vi "CUNNINGHAM_Final-Project_Metal_Foam_Testing.vi"() -> ()   [LabVIEW 2010]
uses:
  <vilib>/Utility/error.llb/DialogType.ctl
  <vilib>/DAQmx/write.llb/DAQmx Write (Analog DBL 1Chan 1Samp).vi
  <vilib>/DAQmx/read.llb/DAQmx Read (Analog Wfm 1Chan NSamp).vi
  <vilib>/DAQmx/read.llb/DAQmx Read (Counter DBL 1Chan 1Samp).vi
  <vilib>/DAQmx/create/channels.llb/DAQmx Create Channel (CI-Frequency).vi
  <vilib>/DAQmx/create/channels.llb/DAQmx Create Channel (AI-Voltage-Basic).vi
  <vilib>/DAQmx/configure/timing.llb/DAQmx Timing (Sample Clock).vi
  <vilib>/DAQmx/create/channels.llb/DAQmx Create Channel (AO-Voltage-Basic).vi
  <vilib>/Utility/file.llb/Write To Spreadsheet File (string).vi
  <vilib>/Utility/file.llb/Write To Spreadsheet File (DBL).vi
  <vilib>/daqmx/miscellaneous.llb/DAQmx Fill In Error Info.vi
  <vilib>/Analysis/NI_AALBase.lvlib
panel:
  out "Collected Data":cluster{"mean":dbl, "data":dbl}[](graph)
  in  "Maximum Value":dbl=10.0 caption="Maximum Voltage to Blower" min=0.0 max=10.0 format="%0.2f"
  in  "Minimum Value":dbl caption="Minimum Voltage to Blower" min=0.0 max=10.0 format="%0.2f"
  out "Current Air Flow Speed (fpm)":dbl
  out "Current Pressure Drop (Pa)":dbl
  out "Frequency (Hz)":dbl format="%0.9f"
  out "Measurement":waveform(dbl)(graph)
  in  "Hold Time(ms)":u32=3000
  in  "Divisions for Air Flow Sweep":u8=5
  in  "Highest Voltage to Blower":dbl=3.3 min=0.0 max=10.0 format="%0.2f"
  in  "Staring Voltage to Blower":dbl=1.3 caption="Starting/Lowest Voltage to Blower" min=0.0 max=10.0 format="%0.2f"
  in  "Physical Channel":tag="Dev1/ao0" caption="AO Physical Channel Output"
  out "Voltage Output":dbl(slide)=1.0 scale=-10.0..9.995 scale format="%.3f"
  in  "AI Maximum Value":dbl=5.0 format="%0.2f"
  in  "AI Minimum Value":dbl format="%0.2f"
  in  "Rate":dbl=1000.0 caption="Sample Rate (Hz)" format="%0.0f"
  in  "Samples per Channel":i32=1000
  in  "Physical Channel":tag="Dev1/ai0" caption="AI Physical Channel Input"
  in  "Minimum Value (Hz)":dbl=1.192093 format="%0.6f"
  in  "Maximum Value (Hz)":dbl=10000000.0 format="%0.6f"
  in  "Edge":i32(ring)=10280 items=["Rising"=10280, "Falling"=10171]
  in  "Counter(s)":tag="Dev1/ctr0" caption="Frequency Physical Channel"
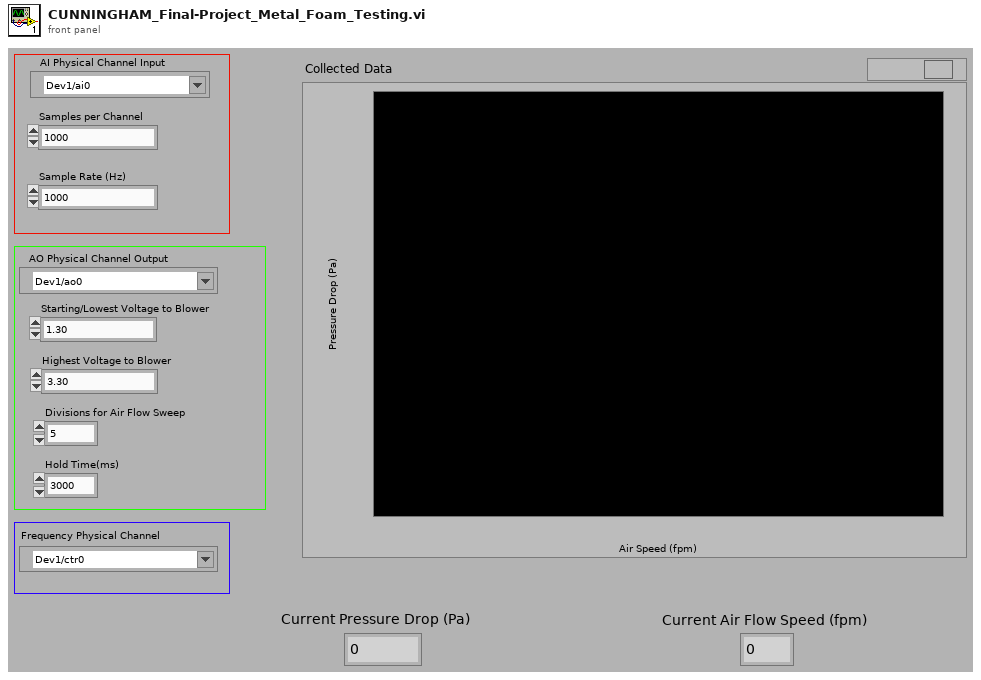
[diagram p1: front panel]
types:
  T1 = typedef "DialogType.ctl" = u16
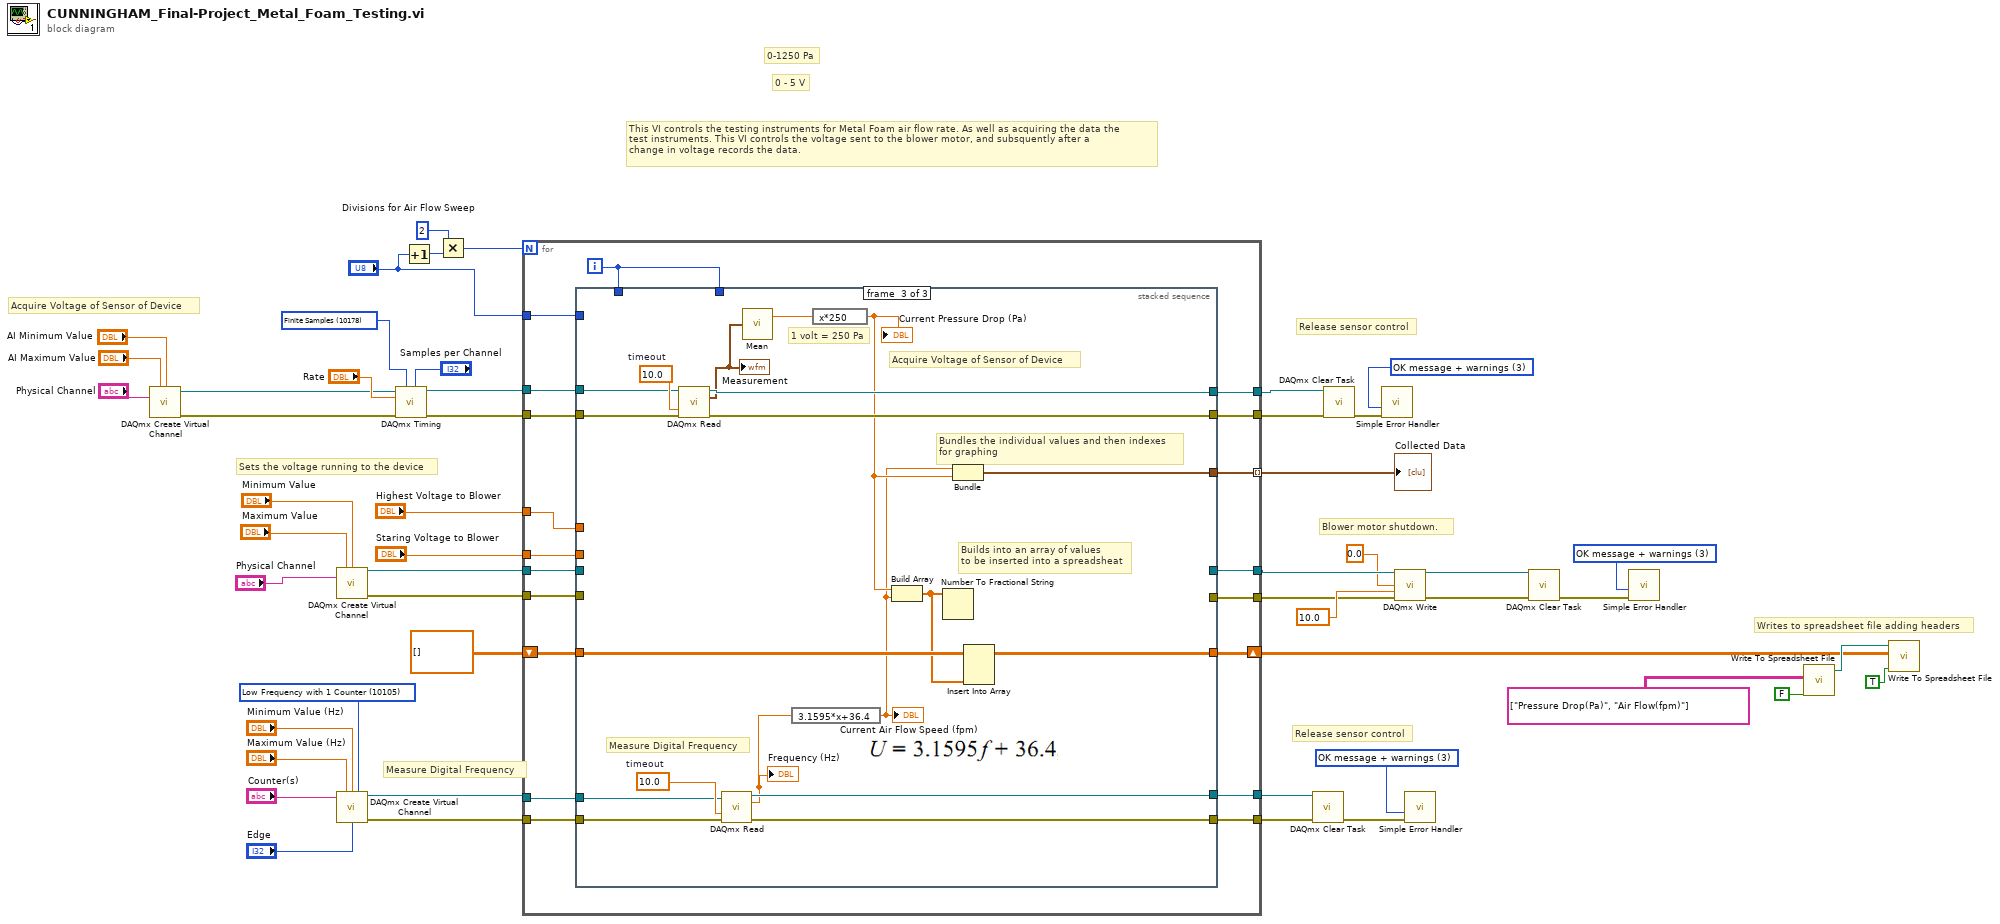
[diagram p0: block diagram]
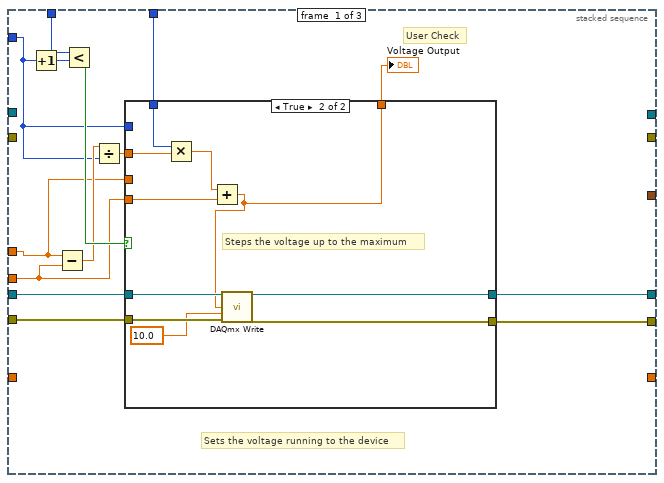
[diagram p2: hidden frame]
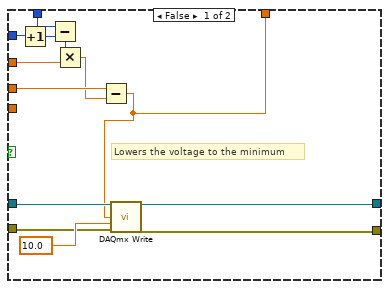
[diagram p3: hidden frame]
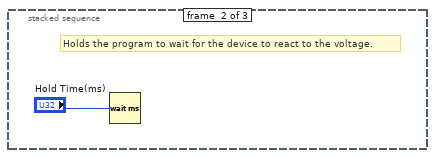
[diagram p4: hidden frame]
diagram:
  w33 = T1 3 items=["no dialog", "OK message", "continue or stop message", "OK message + warnings", "continue/stop + warnings"] ("type of dialog (OK msg:1)")
  w2 = 10178 items=["Finite Samples"=10178, "Continuous Samples"=10123] ("sample mode")
  w44 = T1 3 items=["no dialog", "OK message", "continue or stop message", "OK message + warnings", "continue/stop + warnings"] ("type of dialog (OK msg:1)")
  w49 = 10105 items=["Low Frequency with 1 Counter"=10105, "High Frequency with 2 Counters"=10157, "Large Range with 2 Counters"=10205] ("measurement method")
  w50 = T1 3 items=["no dialog", "OK message", "continue or stop message", "OK message + warnings", "continue/stop + warnings"] ("type of dialog (OK msg:1)")
  # "Writes to spreadsheet file adding headers"
  # "Release sensor control"
  # "Release sensor control"
  # "Sets the voltage running to the device"
  # "0 - 5 V"
  # "0-1250 Pa"
  # "Acquire Voltage of Sensor of Device"
  # "This VI controls the testing instruments for Metal Foam air flow rate. As well as acquiring the data the\ntest instruments. This VI controls the voltage sent to the blower motor, and subsquently after a\nchange in voltage records the data."
  # "Measure Digital Frequency"
  # "Blower motor shutdown."
  n1 = call-poly <vilib>:"DAQmx Create Virtual Channel.vi"("maximum value"="AI Maximum Value", "minimum value"="AI Minimum Value", "physical channels"="Physical Channel") -> ("task out"=w37:refnum<k21>, "error out"=w40:errorcluster)  [unwired: 11 in]
  n2 = call-poly <vilib>:"DAQmx Create Virtual Channel.vi"("maximum value"="Maximum Value", "minimum value"="Minimum Value", "physical channels"="Physical Channel") -> ("task out"=w32:refnum<k21>, "error out"=w30:errorcluster)  [unwired: 11 in]
  n3 = call-poly <vilib>:"DAQmx Create Virtual Channel.vi"("maximum value"="Maximum Value (Hz)", "minimum value"="Minimum Value (Hz)", "measurement method"=w49, "counter"="Counter(s)", "starting edge"="Edge") -> ("task out"=w29:refnum<k21>, "error out"=w28:errorcluster)  [unwired: 9 in]
  n4 = call-poly <vilib>:"DAQmx Timing.vi"("task/channels in"=w37, "sample mode"=w2, "samples per channel"="Samples per Channel", "rate"="Rate", "error in"=w40) -> ("task out"=w35:refnum<k21>, "error out"=w34:errorcluster)  [unwired: 9 in]
  n5 = Increment(x="Divisions for Air Flow Sweep") -> (x+1=w10:u8)
  n6 = Multiply(x=u8 2, y=w10) -> (x*y=w14:u8)
  n7 = for {
    N: w14 -> [_]
    tunnel: w35 -> [w66]
    tunnel: w34 -> [w65]
    tunnel: w32 -> [w70]
    tunnel: [w69] -> w21
    tunnel: [w68] -> w22
    tunnel: w30 -> [w67]
    tunnel: w29 -> [w64]
    tunnel: w28 -> [w63]
    tunnel: [w62] -> w27
    tunnel: [w61] -> w26
    tunnel: [w60] -> w25
    tunnel: [w59] -> w9
    tunnel: "Staring Voltage to Blower" -> [w58]
    tunnel: "Divisions for Air Flow Sweep" -> [w57]
    tunnel: "Highest Voltage to Blower" -> [w56]
    shift-right: [w53] -> w4
    shift-left: dbl[][] [] -> [w54]
    tunnel: [w52] -> w3 mode=indexing
    i -> [w55]
    n8 = stacked-sequence {
      tunnel: w70 -> [w84 _ _]
      tunnel: [w83 _ _] -> w69
      tunnel: [w82 _ _] -> w68
      tunnel: w67 -> [w81 _ _]
      tunnel: w66 -> [_ _ w126]
      tunnel: w65 -> [_ _ w123]
      tunnel: w64 -> [_ _ w121]
      tunnel: w63 -> [_ _ w120]
      tunnel: [_ _ w119] -> w62
      tunnel: [_ _ w118] -> w61
      tunnel: [_ _ w125] -> w60
      tunnel: [_ _ w124] -> w59
      tunnel: w58 -> [w71 _ _]
      tunnel: w57 -> [w73 _ _]
      tunnel: w56 -> [w72 _ _]
      tunnel: w55 -> [w80 _ _]
      tunnel: w55 -> [w78 _ _]
      tunnel: w54 -> [_ _ w114]
      tunnel: [_ _ w112] -> w53
      tunnel: [_ _ w111] -> w52
      frame #0 {
        # "User Check"
        # "Sets the voltage running to the device"
        n9 = Increment(x=w73) -> (x+1=w74:u8)
        n10 = Subtract(x=w72, y=w71) -> (x-y=w76:dbl)
        n11 = Less?(x=w78, y=w74) -> (x < y?=w77:bool)
        n12 = Divide(x=w76, y=w73) -> (x/y=w79:dbl)
        n13 = case shown="True" w77 {
          tunnel: w84 -> [w93 w107]
          tunnel: [w96 w106] -> w83
          tunnel: [w95 w105] -> w82
          tunnel: w81 -> [w94 w104]
          tunnel: w80 -> [w87 w102]
          tunnel: w79 -> [w92 w101]
          tunnel: w71 -> [_ w100]
          tunnel: w73 -> [w85 _]
          tunnel: w72 -> [w90 _]
          tunnel: [w88 w98] -> w75
          frame False {
            # "Lowers the voltage to the minimum"
            n14 = Increment(x=w85) -> (x+1=w86:u8)
            n15 = Subtract(x=w87, y=w86) -> (x-y=w91:i32)
            n16 = Multiply(x=w91, y=w92) -> (x*y=w89:dbl)
            n17 = Subtract(x=w90, y=w89) -> (x-y=w88:dbl)
            n18 = call-poly <vilib>:"DAQmx Write.vi"("task/channels in"=w93, "data"=w88, "timeout"=10.0, "error in"=w94) -> ("task out"=w96:refnum<k21>, "error out"=w95:errorcluster)  [unwired: 9 in, 1 out]
          }
          frame True {
            # "Steps the voltage up to the maximum"
            n19 = Multiply(x=w102, y=w101) -> (x*y=w99:dbl)
            n20 = Add(x=w99, y=w100) -> (x+y=w98:dbl)
            n21 = call-poly <vilib>:"DAQmx Write.vi"("task/channels in"=w107, "data"=w98, "timeout"=10.0, "error in"=w104) -> ("task out"=w106:refnum<k21>, "error out"=w105:errorcluster)  [unwired: 9 in, 1 out]
          }
        }
        "Voltage Output" <- w75
      }
      frame #1 {
        # "Holds the program to wait for the device to react to the voltage."
        n22 = Wait (ms)(milliseconds to wait="Hold Time(ms)") -> ()  [unwired: 1 out]
      }
      frame #2 {
        w122 = 10.0  # timeout
        w127 = 10.0  # timeout
        # "1 volt = 250 Pa"
        # "Bundles the individual values and then indexes\nfor graphing"
        # "Builds into an array of values \nto be inserted into a spreadsheat"
        # "Acquire Voltage of Sensor of Device"
        # "Measure Digital Frequency"
        n23 = call-poly <vilib>:"DAQmx Read.vi"("task/channels in"=w126, "timeout"=w127, "error in"=w123) -> ("task out"=w125:refnum<k21>, "data"=w117:waveform(dbl), "error out"=w124:errorcluster)  [unwired: 10 in]
        "Measurement" <- w117
        n24 = call-poly <vilib>:"DAQmx Read.vi"("task/channels in"=w121, "timeout"=w122, "error in"=w120) -> ("task out"=w119:refnum<k21>, "data"=w115:dbl, "error out"=w118:errorcluster)  [unwired: 10 in]
        "Frequency (Hz)" <- w115
        n25 = call <vilib>:"Mean.vi"("X"=w117) -> ("mean"=w116:dbl)  [unwired: 1 out]
        n26 = expression code="3.1595*x+36.4"(w115) -> (w109:dbl)
        "Current Air Flow Speed (fpm)" <- w109
        n27 = expression code="x*250"(w116) -> (w110:dbl)
        "Current Pressure Drop (Pa)" <- w110
        n28 = Build Array(w110, w109) -> (w113:dbl[])
        n29 = Number To Fractional String(number=w113) -> ()  [unwired: 3 in, 1 out]
        n30 = Bundle("data"=w109, "mean"=w110) -> (w111:cluster{"data":dbl, "mean":dbl})  [unwired: 1 in]
        n31 = Insert Into Array(array=w114, new element=w113) -> (w112:dbl[][])  [unwired: 2 in]
      }
    }
  }
  "Collected Data" <- w3
  n32 = call <vilib>:"DAQmx Clear Task.vi"("task in"=w27, "error in"=w26) -> ("error out"=w43:errorcluster)  [unwired: 13 in]
  n33 = call <vilib>:"DAQmx Clear Task.vi"("task in"=w25, "error in"=w9) -> ("error out"=w39:errorcluster)  [unwired: 13 in]
  n34 = call <vilib>:"Simple Error Handler.vi"("type of dialog (OK msg:1)"=w33, "error in (no error)"=w39) -> ()  [unwired: 3 in, 5 out]
  n35 = call-poly <vilib>:"DAQmx Write.vi"("task/channels in"=w21, "data"=0.0, "timeout"=10.0, "error in"=w22) -> ("task out"=w20:refnum<k21>, "error out"=w19:errorcluster)  [unwired: 9 in, 1 out]
  n36 = call <vilib>:"Simple Error Handler.vi"("type of dialog (OK msg:1)"=w44, "error in (no error)"=w43) -> ()  [unwired: 3 in, 5 out]
  n37 = call <vilib>:"DAQmx Clear Task.vi"("task in"=w20, "error in"=w19) -> ("error out"=w31:errorcluster)  [unwired: 13 in]
  n38 = call <vilib>:"Simple Error Handler.vi"("type of dialog (OK msg:1)"=w50, "error in (no error)"=w31) -> ()  [unwired: 3 in, 5 out]
  n39 = call-poly <vilib>:"Write To Spreadsheet File.vi"("append to file? (new file:F)"=FALSE ("transpose? (no:F)"), "2D data"=string[][] [["Pressure Drop(Pa)", "Air Flow(fpm)"]]) -> ("new file path (Not A Path if cancelled)"=w6:path)  [unwired: 6 in]
  n40 = call-poly <vilib>:"Write To Spreadsheet File.vi"("append to file? (new file:F)"=TRUE, "2D data"=w4, "file path (dialog if empty)"=w6) -> ()  [unwired: 5 in, 1 out]
